vi "Sierra - Frequency Drift test 2-25.vi"() -> ()   [LabVIEW 2015]
doc: "This VI demonstrates a simple procedure for setting up a spectrum analyzer, running an acquisition, and retrieving and plotting the waveform data.\n\nString indicators Binary WF Data and Sgl Float WF Data are initialized to empty strings. Waveform Graph is initialized to 0 for 100000 locations (just an arbitrary number for demonstration purposes).\n\ntkrsa6100 Initialize.vi opens the VISA Resource Name from the information entered by the user. It also presets the instrument by default to the Spectrum measurement. On completion it passes dup VISA Resource Name and error out to the following drivers.\n\nThe next VI to execute is tkrsa6100 Config Frequency.vi. Numeric control Center Freq (MHz)(50) is passed to the VI to set the center frequency to the default 50MHz value. The Set/Read Freq Setting (Set) is not wired since it defaults to SET, which is what is desired in this case. This is the case for all the configuration VI's in the example.\n\nThe next VI to execute is tkrsa6100 Config Spectrum Settings.vi. Enumerated control Spectrum Settings (CENTER FREQUENCY) is passed a Frequency Span constant and numeric control Freq Span (MHz) (40) to set the span to 40MHz.\n\nNext the reference level is set using tkrsa6100 Config RF Input.vi. Enumerated control Input Setting (REFERENCE LEVEL) is passed a Reference Level constant and numeric control Ref Level (dBm)(0) to set the reference level to 0dBm.\n\nNext the acquisition mode is set to single acquisition using tkrsa6100 Config Acquisition.vi. No parameters are passed since the default setting of this VI sets the acquisition mode to single.\n\nA single acquisition is then performed using tkrsa6100 Run Single Acquisition.vi. This VI sends an INIT command followed by a *OPC? Query. When the acquisition is completed the instrument returns a 1 and the next vi executes.\n\nThe binary waveform data is then retrieved by tkrsa6100 Spectrum Msmt Results.vi. The last acquisition data is retrieved by passing constant GET LAST ACQUISITION RESULT to enumerated input Run Acquisition and/or Get Result (RUN ACQUISITION & GET RESULT). The binary data is converted to a comma separated list of single precision floating point numbers by passing constant YES to enumerated input Convert Resp String (NO). The number of display points (total number of data bytes/4) is passed to a Spectral Display property node to scale the x axis of the graph. The binary data string from output Measurement Response String is copied to string indicator Binary WF Data. The converted binary data from output Converted Sgl Float Response String is copied to string indicator Sgl Float WF Data.\n\nSgl Float WF Data is then converted to an array by function Spreadsheet String to Array using a comma as the data separator. The output array is then passed to waveform graph Spectral Display for viewing.\n\nThe VISA Resource Name is closed using tkrsa6100 Close.vi."
panel:
  out "x-y":dbl[][](array[numeric])
  out "Marker\nResponse String 2":string
  out "Marker\nResponse String":string
  in  "Trig Level (dBm)":dbl=-10.0 min=-170.0 max=50.0 step=0.1
  in  "Ref Level (dBm)(0)":dbl min=-170.0 max=50.0 step=0.1
  in  "Msmt Freq (MHz)":dbl=1000.0 min=0.009 max=20000.0 step=1e-06 format="%.6f"
  in  "VISA Resource Name":refnum<visa-resource-name>
  out "Sgl Float WF Data":string
  out "Binary WF Data":string
  out "Spectral Display":dbl[](graph)
  out "error out":errorcluster {"code" format="%#.0f"}
  # "RSA6106A/6114A Acquire and Fetch\nSpectral Analysis Display"
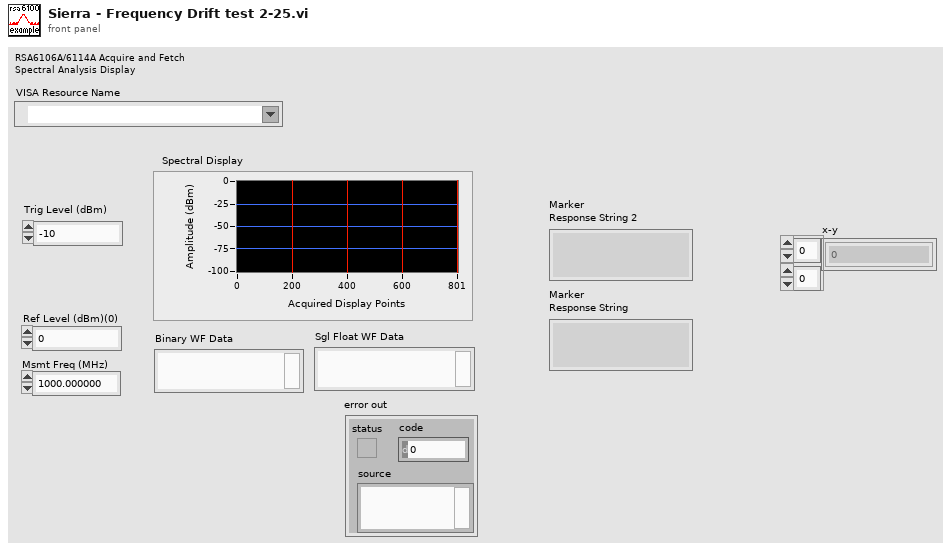
[diagram p1: front panel]
types:
  T1 = enum16{"CENTER FREQUENCY", "FREQUENCY SPAN", "RESOLUTION BW", "MAX REAL TIME SPAN (SET)", "START FREQUENCY", "STOP FREQUENCY", "FREQ STEP SIZE", "AUTO FREQ STEP ON", "AUTO FREQ STEP OFF", "AUTO RES BW ON", "AUTO RES BW OFF", "FFT WINDOW TYPE", "# POINTS", "RBW PROCESS ON", "RBW PROCESS OFF", "GAIN/BW OPTIMIZATION"}
  T2 = enum16{"PEAK FIND (SET)", "NEXT PEAK LOWER (SET)", "NEXT PEAK HIGHER (SET)", "NEXT PEAK LEFT (SET)", "NEXT PEAK RIGHT (SET)", "MARKER TO CF (SET)", "MARKER TO TRACE", "MARKER FREQ", "MARKER AMPL (READ)", "DELTA MARKER FREQ (READ)", "DELTA MARKER AMPL (READ)"}
  T3 = enum16{"RUN ACQUISITION  & GET RESULT", "GET LAST ACQUISITION RESULT"}
  T4 = enum16{"ANALYSIS REFERENCE", "ANALYSIS LENGTH", "ACTUAL ANALYSIS LENGTH (READ)", "AUTO ANALYSIS LENGTH ON", "AUTO ANALYSIS LENGTH OFF", "ANALYSIS OFFSET", "AUTO ANALYSIS OFFSET ON", "AUTO ANALYSIS OFFSET OFF", "SPECTRUM LENGTH", "ACTUAL SPECTRUM LENGTH (READ)", "AUTO SPECTRUM LENGTH ON", "AUTO SPECTRUM LENGTH OFF", "SPECTRUM OFFSET", "SPECTRUM TIME MODE", "DITHER MODE", "DITHER HW STATUS (READ)", "AUTO SPECTRUM OFFSETS AND ANALYSIS"}
  T5 = enum16{"TRIGGER SOURCE", "TRIGGER ON", "TRIGGER OFF", "TIME DELAY", "TIME POSITION", "TRIGGER EACH SEGMENT ON", "TRIGGER EACH SEGMENT OFF", "TRIGGER TYPE POWER", "TRIGGER TYPE FREQ MASK", "TRIGGER LEVEL", "TRIGGER SLOPE RISING", "TRIGGER SLOPE FALLING", "TDBW MODE ON", "TDBW MODE OFF", "TDBW", "ACTUAL TDBW (READ)", "CREATE NEW FMT (SET)", "SAVE FMT (SET)", "LOAD FMT (SET)", "FMT VIOLATION LOGIC", "FMT RBW AUTO", "FMT RBW MANUAL", "FMT RBW", "FORCE TRIGGER", "Trigger Position Auto"}
  T6 = enum16{"SPECTRUM ANALYZER", "DPSA", "SPECTROGRAM", "AMPL VS TIME", "FREQ VS TIME", "PHASE VS TIME", "IQ VS TIME", "TIME OVERVIEW"}
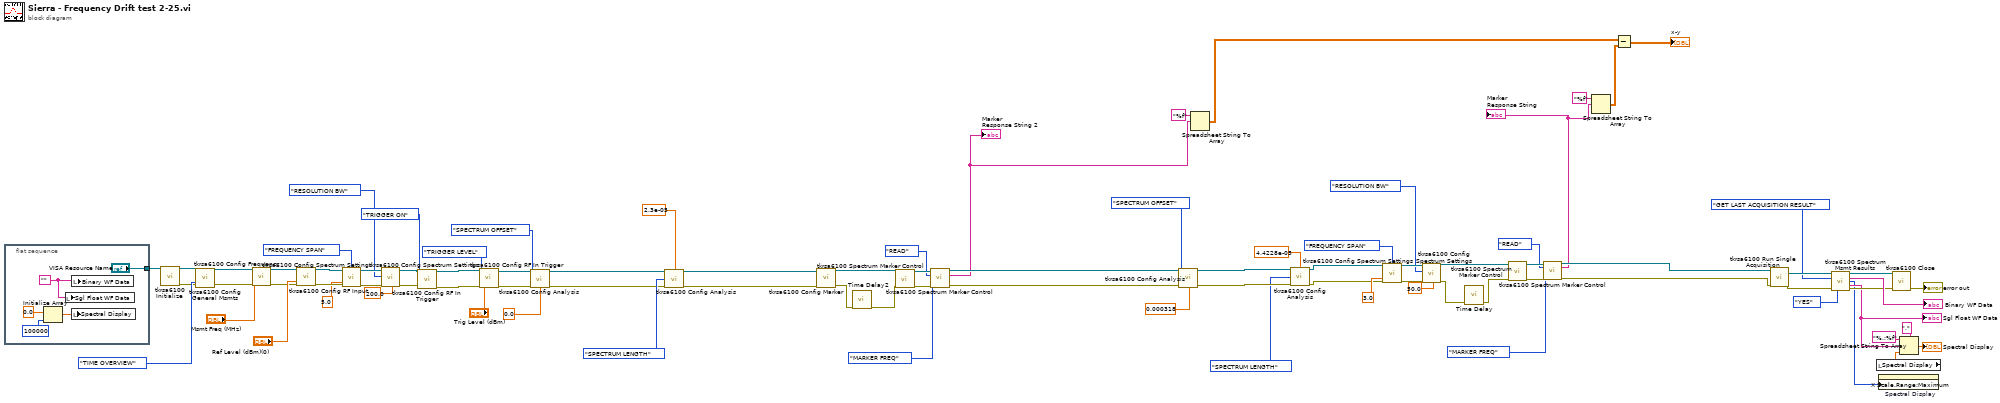
[diagram p0: block diagram]
diagram:
  n1 = flat-sequence {
    tunnel: ["VISA Resource Name"] -> w78
    frame #0 {
      w90 = ""
      n2 = Initialize Array(0.0 ("element"), 100000 ("dimension size")) -> (w92:dbl[])
      n3 = local write "Sgl Float WF Data"(w90) -> ()
      n4 = local write "Spectral Display"(w92) -> ()
      n5 = local write "Binary WF Data"(w90) -> ()
    }
  }
  n6 = call <instrlib>:"tkrsa6100 Initialize.vi"("VISA Resource Name"=w78) -> ("dup VISA Resource Name"=w74:refnum<visa-resource-name>, "error out"=w75:errorcluster)  [unwired: 3 in, 10 out]
  n7 = call <instrlib>:"tkrsa6100 Config General Msmts.vi"("VISA Resource Name"=w74, "Measurement\n(SPECTRUM ANALYZER)"=T6."TIME OVERVIEW" ("Measurement\n(SPECTRUM ANALYZER)"), "error in (no error)"=w75) -> ("dup VISA Resource Name"=w55:refnum<visa-resource-name>, "error out"=w54:errorcluster)  [unwired: 10 in, 1 out]
  n8 = call <instrlib>:"tkrsa6100 Config Frequency.vi"("VISA Resource Name"=w55, "Msmt Freq (MHz)\n(1000)"="Msmt Freq (MHz)", "error in (no error)"=w54) -> ("dup VISA Resource Name"=w53:refnum<visa-resource-name>, "error out"=w52:errorcluster)  [unwired: 1 in, 10 out]
  n9 = call <instrlib>:"tkrsa6100 Config RF Input.vi"("VISA Resource Name"=w53, "Ref Level (0)"="Ref Level (dBm)(0)", "error in (no error)"=w52) -> ("dup VISA Resource Name"=w45:refnum<visa-resource-name>, "error out"=w44:errorcluster)  [unwired: 4 in, 7 out]
  n10 = call <instrlib>:"tkrsa6100 Config Spectrum Settings.vi"("VISA Resource Name"=w45, "Spectrum Settings\n (CENTER FREQUENCY)"=T1."FREQUENCY SPAN" ("Spectrum Settings\n (CENTER FREQUENCY)"), "Freq Span\n(MHz)(40)"=5.0 ("Freq Span\n(MHz)(40)"), "error in (no error)"=w44) -> ("dup VISA Resource Name"=w35:refnum<visa-resource-name>, "error out"=w34:errorcluster)  [unwired: 13 in, 1 out]
  n11 = call <instrlib>:"tkrsa6100 Config Spectrum Settings.vi"("VISA Resource Name"=w35, "Spectrum Settings\n (CENTER FREQUENCY)"=T1."RESOLUTION BW" ("Spectrum Settings\n (CENTER FREQUENCY)"), "error in (no error)"=w34, "Res BW (KHz)\n(300)"=200.0 ("Res BW (KHz)\n(300)")) -> ("dup VISA Resource Name"=w33:refnum<visa-resource-name>, "error out"=w32:errorcluster)  [unwired: 13 in, 1 out]
  n12 = call <instrlib>:"tkrsa6100 Config RF In Trigger.vi"("VISA Resource Name"=w33, "Trigger Settings\n(TRIGGER SOURCE)"=T5."TRIGGER ON" ("Trigger Settings\n(TRIGGER SOURCE)"), "error in (no error)"=w32) -> ("dup VISA Resource Name"=w60:refnum<visa-resource-name>, "error out"=w61:errorcluster)  [unwired: 14 in, 1 out]
  n13 = call <instrlib>:"tkrsa6100 Config RF In Trigger.vi"("VISA Resource Name"=w60, "Trigger Settings\n(TRIGGER SOURCE)"=T5."TRIGGER LEVEL" ("Trigger Settings\n(TRIGGER SOURCE)"), "error in (no error)"=w61, "Trig Level\n(dBm)(-10)"="Trig Level (dBm)") -> ("dup VISA Resource Name"=w41:refnum<visa-resource-name>, "error out"=w40:errorcluster)  [unwired: 13 in, 1 out]
  n14 = call <instrlib>:"tkrsa6100 Config Analysis.vi"("VISA Resource Name"=w41, "Analysis Setting\n(ANALYSIS REFERENCE)"=T4."SPECTRUM OFFSET" ("Analysis Setting\n(ANALYSIS REFERENCE)"), "error in (no error)"=w40, "Offset Tme (S)(0)"=0.0) -> ("dup VISA Resource Name"=w58:refnum<visa-resource-name>, "error out"=w59:errorcluster)  [unwired: 9 in, 1 out]
  n15 = call <instrlib>:"tkrsa6100 Config Analysis.vi"("VISA Resource Name"=w58, "Length (S)(0.022)"=2.3e-05, "Analysis Setting\n(ANALYSIS REFERENCE)"=T4."SPECTRUM LENGTH" ("Analysis Setting\n(ANALYSIS REFERENCE)"), "error in (no error)"=w59) -> ("dup VISA Resource Name"=w22:refnum<visa-resource-name>, "error out"=w21:errorcluster)  [unwired: 9 in, 1 out]
  n16 = call <instrlib>:"tkrsa6100 Config Marker.vi"("VISA Resource Name"=w22, "error in (no error)"=w21) -> ("dup VISA Resource Name"=w29:refnum<visa-resource-name>, "error out"=w25:errorcluster)  [unwired: 11 in, 1 out]
  n17 = call "Time Delay2"("error in (no error)"=w25) -> ("error out"=w24:errorcluster)  [unwired: 10 in]
  n18 = call <instrlib>:"tkrsa6100 Spectrum Marker Control.vi"("VISA Resource Name"=w29, "error in (no error)"=w24) -> ("dup VISA Resource Name"=w28:refnum<visa-resource-name>, "error out"=w27:errorcluster)  [unwired: 11 in, 1 out]
  n19 = call <instrlib>:"tkrsa6100 Spectrum Marker Control.vi"("VISA Resource Name"=w28, "Set/Read\nMarker Functions (SET)"=enum16{"SET", "READ"}."READ" ("Set/Read\nMarker Functions (SET)"), "Marker Function\n(PEAK FIND)"=T2."MARKER FREQ" ("Marker Function\n(PEAK FIND)"), "error in (no error)"=w27) -> ("dup VISA Resource Name"=w20:refnum<visa-resource-name>, "Marker\nResponse String"=w18:string, "error out"=w19:errorcluster)  [unwired: 9 in]
  "Marker\nResponse String 2" <- w18
  n20 = call <instrlib>:"tkrsa6100 Config Analysis.vi"("VISA Resource Name"=w20, "Analysis Setting\n(ANALYSIS REFERENCE)"=T4."SPECTRUM OFFSET" ("Analysis Setting\n(ANALYSIS REFERENCE)"), "error in (no error)"=w19, "Offset Tme (S)(0)"=0.000318) -> ("dup VISA Resource Name"=w49:refnum<visa-resource-name>, "error out"=w48:errorcluster)  [unwired: 9 in, 1 out]
  n21 = Spreadsheet String To Array(format string="%f", spreadsheet string=w18) -> (array=w16:dbl[][])  [unwired: 2 in]
  n22 = call <instrlib>:"tkrsa6100 Config Analysis.vi"("VISA Resource Name"=w49, "Length (S)(0.022)"=4.4228e-05, "Analysis Setting\n(ANALYSIS REFERENCE)"=T4."SPECTRUM LENGTH" ("Analysis Setting\n(ANALYSIS REFERENCE)"), "error in (no error)"=w48) -> ("dup VISA Resource Name"=w5:refnum<visa-resource-name>, "error out"=w4:errorcluster)  [unwired: 9 in, 1 out]
  n23 = call <instrlib>:"tkrsa6100 Config Spectrum Settings.vi"("VISA Resource Name"=w5, "Spectrum Settings\n (CENTER FREQUENCY)"=T1."FREQUENCY SPAN" ("Spectrum Settings\n (CENTER FREQUENCY)"), "Freq Span\n(MHz)(40)"=3.0 ("Freq Span\n(MHz)(40)"), "error in (no error)"=w4) -> ("dup VISA Resource Name"=w9:refnum<visa-resource-name>, "error out"=w8:errorcluster)  [unwired: 13 in, 1 out]
  n24 = call <instrlib>:"tkrsa6100 Config Spectrum Settings.vi"("VISA Resource Name"=w9, "Spectrum Settings\n (CENTER FREQUENCY)"=T1."RESOLUTION BW" ("Spectrum Settings\n (CENTER FREQUENCY)"), "error in (no error)"=w8, "Res BW (KHz)\n(300)"=50.0 ("Res BW (KHz)\n(300)")) -> ("dup VISA Resource Name"=w3:refnum<visa-resource-name>, "error out"=w2:errorcluster)  [unwired: 13 in, 1 out]
  n25 = call "Time Delay"("error in (no error)"=w2) -> ("error out"=w1:errorcluster)  [unwired: 10 in]
  n26 = call <instrlib>:"tkrsa6100 Spectrum Marker Control.vi"("VISA Resource Name"=w3, "error in (no error)"=w1) -> ("dup VISA Resource Name"=w66:refnum<visa-resource-name>, "error out"=w65:errorcluster)  [unwired: 11 in, 1 out]
  n27 = call <instrlib>:"tkrsa6100 Spectrum Marker Control.vi"("VISA Resource Name"=w66, "Set/Read\nMarker Functions (SET)"=enum16{"SET", "READ"}."READ" ("Set/Read\nMarker Functions (SET)"), "Marker Function\n(PEAK FIND)"=T2."MARKER FREQ" ("Marker Function\n(PEAK FIND)"), "error in (no error)"=w65) -> ("dup VISA Resource Name"=w38:refnum<visa-resource-name>, "Marker\nResponse String"=w14:string, "error out"=w37:errorcluster)  [unwired: 9 in]
  "Marker\nResponse String" <- w14
  n28 = Spreadsheet String To Array(format string="%f", spreadsheet string=w14) -> (array=w13:dbl[][])  [unwired: 2 in]
  n29 = Subtract(x=w16, y=w13) -> (x-y=→"x-y":dbl[][])
  n30 = call <instrlib>:"tkrsa6100 Run Single Acquisition.vi"("VISA Resource Name"=w38, "error in (no error)"=w37) -> ("dup VISA Resource Name"=w63:refnum<visa-resource-name>, "error out"=w62:errorcluster)  [unwired: 12 out]
  n31 = call <instrlib>:"tkrsa6100 Spectrum Msmt Results.vi"("VISA Resource Name"=w63, "Run Acquisition and/or \nGet Result (RUN ACQUISITION & GET RESULT)"=T3."GET LAST ACQUISITION RESULT" ("Run Acquisition and/or \nGet Result (RUN ACQUISITION & GET RESULT)"), "error in (no error)"=w62, "Convert Resp\nString(NO)"=enum16{"NO", "YES"}."YES" ("Convert Resp\nString(NO)")) -> ("dup VISA Resource Name"=w81:refnum<visa-resource-name>, "Measurement\nResponse String"=→"Binary WF Data":string, "# Data Points"=w79:i32, "Converted Sgl Float\nResponse String"=w80:string, "error out"=w83:errorcluster)  [unwired: 7 in]
  "Sgl Float WF Data" <- w80
  n32 = local read "Spectral Display"() -> (w88:dbl[])
  n33 = property on="Spectral Display" class="WFGraph (strict)"("X Scale.Range:Maximum"=w79) -> ()  [unwired: 2 in, 2 out]
  n34 = call <instrlib>:"tkrsa6100 Close.vi"("VISA Resource Name"=w81, "error in (no error)"=w83) -> ("error out"=→"error out":errorcluster)  [unwired: 13 out]
  n35 = Spreadsheet String To Array(delimiter (Tab)=",", format string="%.;%f", spreadsheet string=w80, array type (2D Dbl)=w88) -> (array=→"Spectral Display":dbl[])
